vi "Get Slave Info.vi"(8 "error in (no error)":errorcluster, 11 "Item Ref in":T1 format="%.0x") -> (0 "error out":errorcluster, 1 "Slave #":u16, 2 "Slave Name":string, 3 "Item Ref out":T1 format="%.0x", 5 "Prepend":bool)   [LabVIEW 2016, in "Scan Engine Custom Device.lvlib"]
uses:
  Scan Engine Custom Device.lvlib
  <vilib>/NI Veristand/Custom Device API/Custom Device Item Ref.ctl
  Globals/Property Strings.vi
  <vilib>/NI Veristand/Custom Device API/Get Item Property (Boolean).vi
  <vilib>/NI Veristand/Custom Device API/Get Item Property (U16).vi
  <vilib>/NI Veristand/Custom Device API/Custom Device API.lvlib
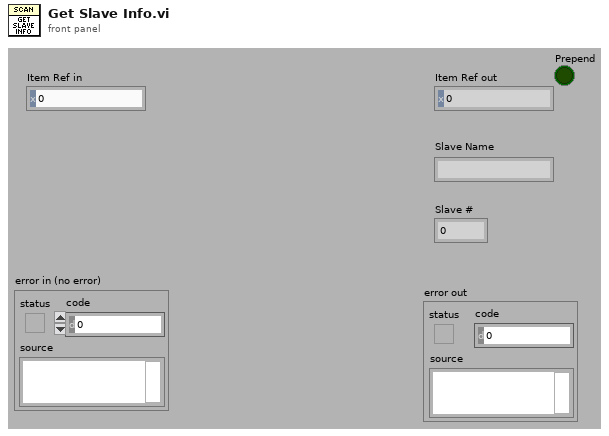
[diagram p1: front panel]
types:
  T1 = typedef "Custom Device API.lvlib/Custom Device Item Ref.ctl" = u64
  T2 = typedef "Custom Device API.lvlib/Custom Device Item Info.ctl" = cluster{"Name":string, "Is Channel":bool, "GUID":string, "Is Waveform":bool}
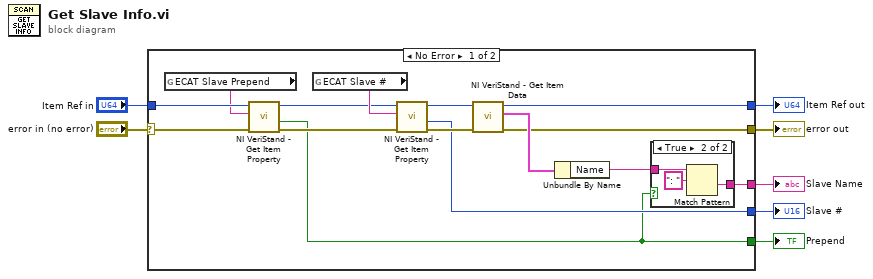
[diagram p0: block diagram]
diagram:
  n1 = case shown="No Error" "error in (no error)" {
    selector: "error in (no error)" -> [w12 w28]
    tunnel: [w16 w28] -> w6
    tunnel: "Item Ref in" -> [w13 w27]
    tunnel: [w17 w27] -> w4
    tunnel: [w15 _] -> w3
    tunnel: [w14 _] -> w2
    tunnel: [w8 _] -> w1
    frame No Error {
      n2 = global read "Property Strings.vi" "ECAT Slave Prepend"() -> (w11:string)
      n3 = call-poly <vilib>:"NI VeriStand - Get Item Property.vi"("error in (no error)"=w12, "Property Name"=w11, "Item Ref in"=w13) -> ("error out"=w9:errorcluster, "Value"=w8:bool, "Item Ref out"=w10:T1)  [unwired: 5 in, 1 out]
      n4 = global read "Property Strings.vi" "ECAT Slave #"() -> (w22:string)
      n5 = call-poly <vilib>:"NI VeriStand - Get Item Property.vi"("error in (no error)"=w9, "Property Name"=w22, "Item Ref in"=w10) -> ("error out"=w18:errorcluster, "Value"=w14:u16, "Item Ref out"=w19:T1)  [unwired: 5 in, 1 out]
      n6 = call <vilib>:"NI VeriStand - Get Item Data.vi"("error in (no error)"=w18, "Item Ref in"=w19) -> ("error out"=w16:errorcluster, "Item Info"=w20:T2, "Item Ref out"=w17:T1)  [unwired: 7 out]
      n7 = Unbundle By Name(w20) -> ("Name"=w21:string)
      n8 = case shown="True" w8 {
        tunnel: w21 -> [w23 w25]
        tunnel: [w23 w24] -> w15
        frame False {
        }
        frame True {
          n9 = Match Pattern(string=w25, regular expression=": " ("search string/char (-)")) -> (after substring=w24:string)  [unwired: 1 in, 3 out]
        }
      }
    }
    frame Error {
    }
  }
  "error out" <- w6
  "Item Ref out" <- w4
  "Slave #" <- w2
  "Slave Name" <- w3
  "Prepend" <- w1
